vi "1_SN Patch file.vi"(9 "CSV path":path=path "D:/20161122/LNK01E-213300ALF/Serial_Log.csv", 10 "PCBA Barcode":string="SVI77664916000894", 11 "Test Operator ID":string="13984") -> (0 "Check SUM HEX":string, 1 "Serial number (Hex)":string, 2 "Logfile":string[][](table), 3 "PCBA Barcode out":string="SVI77664916000894")   [LabVIEW 2018]
panel:
  out "Record Found":bool
  out "Path":path
  in  "input String (Serial Number) 8 Digit":string="5051525354A5A6A7A8A9"
  out "Replace xx with Check sum (Byte5)":string
  out "Replace YYYYYYYY with new serial number( Byte 1 - 4)":string
  out "Input Hex file":string
  in  "Input File":path=path "D:/20161122/LNK01E-213300ALF/Firmware/InputFile.hex"
  # "SVI77664916000895"
  # "SVI77664916000894"
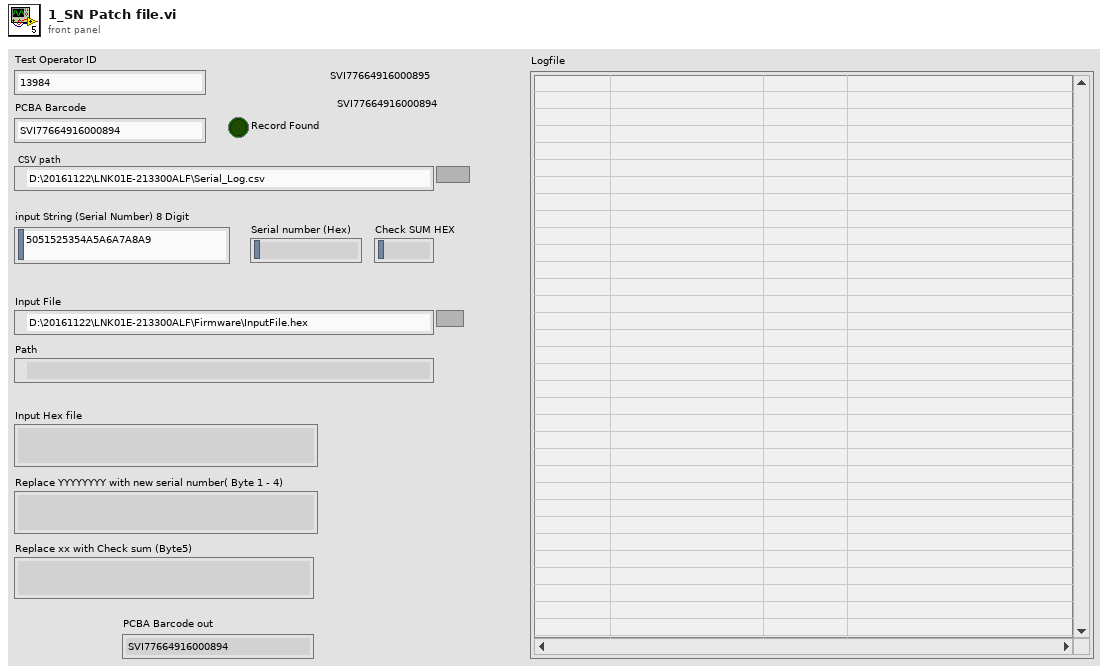
[diagram p1: front panel]
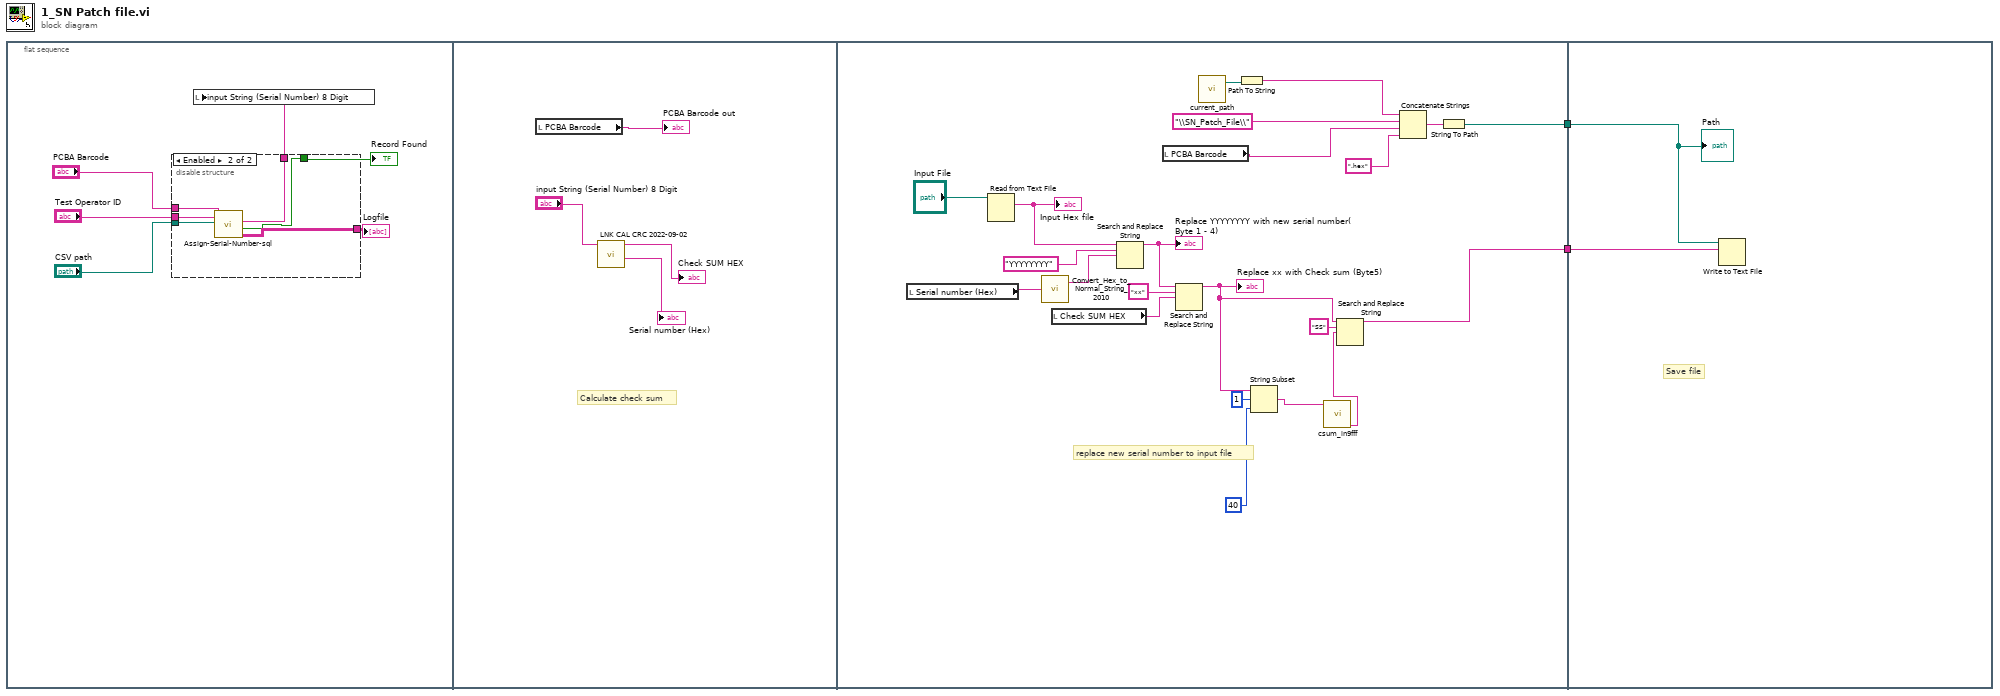
[diagram p0: block diagram]
diagram:
  n1 = flat-sequence {
    tunnel: [w31] -> w2
    tunnel: [w33] -> w1
    tunnel: w2 -> [w48]
    tunnel: w1 -> [w47]
    frame #0 {
      n2 = disable-structure shown="Enabled" {
        disable-tunnel: "PCBA Barcode" -> [w14 w19]
        disable-tunnel: "CSV path" -> [w13 w18]
        disable-tunnel: "Test Operator ID" -> [w12 w20]
        disable-tunnel: [w11 w17] -> w5
        disable-tunnel: [w10 w16] -> w4
        disable-tunnel: [w9 w15] -> w3
        frame Disabled {
        }
        frame Enabled {
          n3 = call "Assign-Serial-Number-sql.vi"("CSV path"=w18, "Test Operator ID"=w20, "PCBA Barcode"=w19) -> ("Table"=w16:string[][], "Record Found"=w15:bool, "Serial Number (STR)"=w17:string)  [unwired: 5 in, 1 out]
        }
      }
      "Logfile" <- w4
      "Record Found" <- w3
      n4 = local write "input String (Serial Number) 8 Digit"(w5) -> ()
    }
    frame #1 {
      # "Calculate check sum"
      n5 = local read "PCBA Barcode"() -> (→"PCBA Barcode out":string)
      n6 = call "LNK CAL CRC 2022-09-02.vi"("Serial number in"="input String (Serial Number) 8 Digit") -> ("Serial number in Hex"=→"Serial number (Hex)":string, "Check SUM HEX"=→"Check SUM HEX":string)  [unwired: 8 in, 1 out]
    }
    frame #2 {
      # "replace new serial number to input file"
      n7 = local read "Serial number (Hex)"() -> (w39:string)
      n8 = Read from Text File(file (use dialog)="Input File") -> (text=w45:string)  [unwired: 3 in, 3 out]
      "Input Hex file" <- w45
      n9 = call "Convert_Hex_to_Normal_String_2010.vi"("Initial Hex String"=w39) -> ("Normal String - Number to Hexadecimal String Method"=w43:string)  [unwired: 1 out]
      n10 = local read "Check SUM HEX"() -> (w40:string)
      n11 = Search and Replace String(input string=w45, search string="YYYYYYYY" ("input string"), replace string=w43) -> (result string=w42:string)  [unwired: 5 in, 3 out]
      "Replace YYYYYYYY with new serial number( Byte 1 - 4)" <- w42
      n12 = local read "PCBA Barcode"() -> (w32:string)
      n13 = Search and Replace String(input string=w42, search string="xx" ("input string"), replace string=w40) -> (result string=w29:string)  [unwired: 5 in, 3 out]
      "Replace xx with Check sum (Byte5)" <- w29
      n14 = call "current_path.vi"() -> ("stripped path"=w38:path)  [unwired: 2 in, 1 out]
      n15 = Path To String(path=w38) -> (string=w37:string)
      n16 = String Subset(string=w29, offset (0)=1, length (rest)=40 ("length (rest)")) -> (substring=w26:string)
      n17 = call "csum_in9fff.vi"("string"=w26) -> ("hex integer string"=w25:string)  [unwired: 9 in, 1 out]
      n18 = Search and Replace String(input string=w29, search string="SS", replace string=w25) -> (result string=w31:string)  [unwired: 5 in, 3 out]
      n19 = Concatenate Strings(w37, "\\SN_Patch_File\\", w32, ".hex") -> (w34:string)
      n20 = String To Path(string=w34) -> (path=w33:path)
    }
    frame #3 {
      # "Save file"
      n21 = Write to Text File(file (use dialog)=w47, text=w48) -> ()  [unwired: 2 in, 3 out]
      "Path" <- w47
    }
  }
